vi "add.sub.to.map.vi"(9 "id":i32, 10 "data":T1[](array[typedef]), 11 "map out":T2) -> (2 "issue map":map{i32, string}(c390), 3 "map out":T2)   [LabVIEW 2024, in "manager_daemon.lvclass"]
uses:
  manager_daemon.lvclass
  type_defs/sub-map--map.ctl
  type_defs/SubData--cluster.ctl
  CV_RESTful_Library/typedefs/cv_issue.generic_credit--cluster.ctl
  manager_daemon.lvclass/manager_daemon.ctl
  CV_RESTful_Library/CV_RESTful_Lib.lvlib
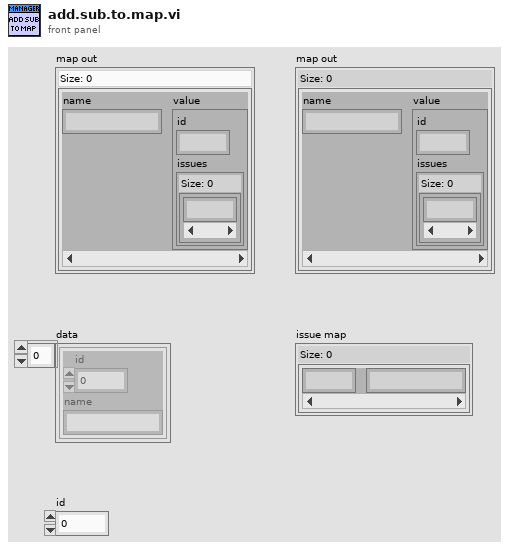
[diagram p1: front panel]
types:
  T1 = typedef "CV_RESTful_Lib.lvlib/cv_issue.generic_credit--cluster.ctl" = cluster{"id":i32, "name":string}
  T2 = typedef "manager_daemon.lvclass/sub-map--map.ctl" = map{string, T3}
  T3 = typedef "manager_daemon.lvclass/SubData--cluster.ctl" = cluster{"id":i32, "issues":set{i32}}
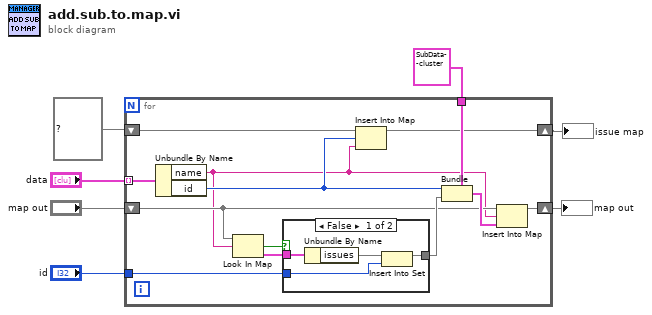
[diagram p0: block diagram]
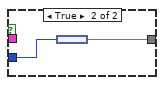
[diagram p2: hidden frame]
diagram:
  n1 = for {
    tunnel: "data" -> [w20] mode=indexing
    shift-right: [w17] -> w7
    shift-left: "map out" -> [w13]
    tunnel: "id" -> [w18]
    tunnel: T3 {"id"=0, "issues"={}} ("output cluster") -> [w12]
    shift-right: [w10] -> w1
    shift-left: map{i32, string} {} ("map") -> [w11]
    n2 = Unbundle By Name(w20) -> ("name"=w8:string, "id"=w9:i32)
    n3 = Look In Map(map=w13, key=w8) -> (key not found?=w19:bool, value=w16:T3)  [unwired: 1 in]
    n4 = case shown="False" w19 {
      tunnel: w18 -> [w22 w26]
      tunnel: w16 -> [w24 _]
      tunnel: [w21 w25] -> w15
      frame False {
        n5 = Unbundle By Name(w24) -> ("issues"=w23:set{i32})
        n6 = Insert Into Set(10:w22, 11:w23) -> (3:w21:set{i32})  [unwired: 1 out]
      }
      frame True {
        n7 = node(w26) -> (w25:set{i32})
      }
    }
    n8 = Insert Into Map(map in=w11, key=w9, value=w8) -> (map out=w10:map{i32, string})  [unwired: 2 out]
    n9 = Bundle(cluster=w12, "id"=w9, "issues"=w15) -> (w14:T3)
    n10 = Insert Into Map(map in=w13, key=w8, value=w14) -> (map out=w17:T2)  [unwired: 2 out]
  }
  "map out" <- w7
  "issue map" <- w1
